vi "get all names.vi"(8 "error in (no error)":errorcluster, 11 "SysObj in":refnum<class "Folder.lvclass">) -> (0 "error out":errorcluster, 2 "Names":path[](array[path]), 3 "SysObj out":refnum<class "Folder.lvclass">)   [LabVIEW 2020, in "Folder.lvclass"]
uses:
  Folder.lvclass
  Folder.lvclass/Folder.ctl
  system object/system object.lvclass
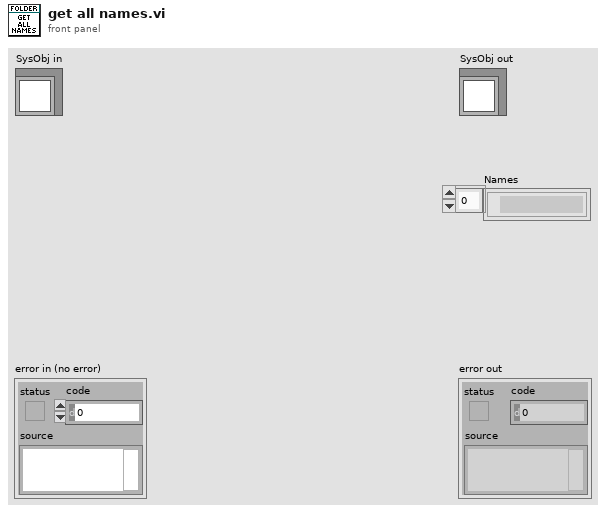
[diagram p1: front panel]
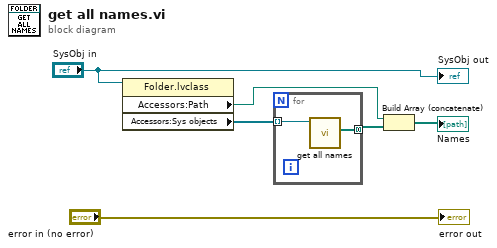
[diagram p0: block diagram]
diagram:
  n1 = property class="Folder.lvclass"(reference="SysObj in") -> ("Accessors:Path"=w3:path, "Accessors:Sys objects"=w5:refnum<class "system object.lvclass">[])  [unwired: 1 in, 2 out]
  n2 = for {
    tunnel: w5 -> [w8] mode=indexing
    tunnel: [w7] -> w4 mode=concatenating
    n3 = call-dynamic "get all names.vi"("SysObj in"=w8) -> ("Names"=w7:path[])  [unwired: 8 in, 2 out]
  }
  n4 = Build Array (concatenate)(w3, w4) -> (→"Names":path[])
  "error out" <- "error in (no error)"
  "SysObj out" <- "SysObj in"
